vi "Enable All Disabled Programs.vi"(11 "EXID":u32=16773121 step=1 format="%.0x") -> ()   [LabVIEW 2010]
doc: "This VI Searches all device programs for programs that are defined AND disabled and re-enables them. This needs to be done to clear the device ActiveError byte."
uses:
  Drivers/Telemetry/Typedef Command List.ctl
panel:
  out "Affected Programs":string
  out "error out":errorcluster
  in  "error in (no error)":errorcluster
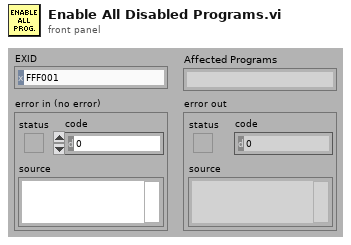
[diagram p1: front panel]
types:
  T1 = enum16{"Open Session", "Close Session", "Downlink Only", "Uplink Only", "Transceive (DN -> UP)"}
  T2 = typedef "Typedef Command List.ctl" = enum16{"Get xPG Status", "xPG Stimulation", "Select Program", "Increment Program Amplitude", "Decrement Program Amplitude", "Get PoP Constants", "Get PPC Constants", "Get Program Names", "Set Pulse Amplitude", "Increment Pulse Amplitude", "Decrement Pulse Amplitude", "Get Pulse Widths", "Set Pulse Widths", "Increment Pulse Width", "Decrement Pulse Width", "Get Program Frequency", "Set Program Frequency", "Increment Program Frequency", "Decrement Program Frequency", "Inject Event", "Charging Control", "Get xPG Identity", "Set xPG Identity", "Restore Program Defaults", "Get Program Definition", "Set Program Definition", "Get Program Constants", "Set Program Constants", "Get Configurable Device Parameters", "Set Configurable Device Parameters", "Get Pulse Constants", "Set Pulse Constants", "Get Lead Limits", "Set Lead Limits", "Get Channel Calibrations", "Set Channel Calibrations", "<reserved 2>", "<reserved 3>", "<reserved 4>", "<reserved 5>", "<reserved 6>", "<reserved 7>", "Get Stim Asic HV Calibrations", "Set Stim Asic HV Calibrations", "<reserved 8>", "<reserved 9>", "Get CP Data", "Set CP Data", "Clear Log", "Read Log", "Append Log", "Get Patient Program Runtime", "Set Patient Program Runtime", "Impedance Measurement", "Enter Storage Mode", "Echo Short", "Echo Long", "Get General Calibration", "Set General Calibration", "Get Trim List", "Set Trim List", "Get Counter", "Set Counter", "Get Test Stimulation", "Set Test Stimulation", "Get Titration Stimulation", "Set Titration Stimulation", "Get Ramp Time", "Set Ramp Time", "Get VBAT", "Set Software Description Block", "Get Software Description Block", "Write Memory", "Read Memory", "Reset xPG", "Erase Flash Block", "Write Vectors", "Read Vectors", "Diagnostic Data", "Set Background Impedance", "Get Background Impedence ", "Undefined"}
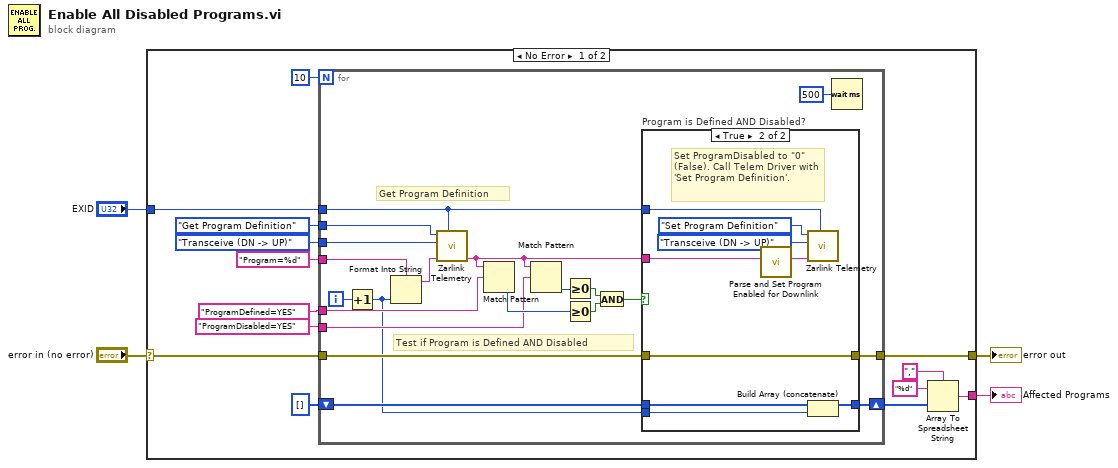
[diagram p0: block diagram]
diagram:
  n1 = case shown="No Error" "error in (no error)" {
    selector: "error in (no error)" -> [w13 w50]
    tunnel: [w12 w50] -> w3
    tunnel: [w6 _] -> w2
    tunnel: "EXID" -> [w5 _]
    frame No Error {
      n2 = for {
        N: 10 -> [_]
        tunnel: Typedef_Command_List."Get Program Definition" ("Command") -> [w38]
        tunnel: T1."Transceive (DN -> UP)" ("Function") -> [w37]
        tunnel: "Program=%d" -> [w35]
        tunnel: "ProgramDefined=YES" ("regular expression") -> [w33]
        tunnel: "ProgramDisabled=YES" ("regular expression") -> [w20]
        tunnel: w13 -> [w26]
        tunnel: [w25] -> w12
        shift-right: [w24] -> w9
        shift-left: i32[] [] -> [w23]
        tunnel: w5 -> [w21]
        i -> [w34]
        # "Test if Program is Defined AND Disabled"
        # "Get Program Definition"
        n3 = Increment(x=w34) -> (x+1=w19:i32)
        n4 = Format Into String(format string=w35, w19) -> (resulting string=w36:string)  [unwired: 2 in, 1 out]
        n5 = call "Zarlink Telemetry.vi"("EXID"=w21, "Parameters"=w36, "Function"=w37, "Command"=w38) -> ("Data"=w27:string)  [unwired: 2 in, 5 out]
        n6 = Match Pattern(string=w27, regular expression=w33) -> (offset past match=w32:i32)  [unwired: 1 in, 3 out]
        n7 = Match Pattern(string=w27, regular expression=w20) -> (offset past match=w31:i32)  [unwired: 1 in, 3 out]
        n8 = Greater Or Equal To 0?(x=w31) -> (x >= 0?=w29:bool)
        n9 = Greater Or Equal To 0?(x=w32) -> (x >= 0?=w30:bool)
        n10 = And(x=w29, y=w30) -> (x .and. y?=w28:bool)
        n11 = case "Program is Defined AND Disabled?" shown="True" w28 {
          tunnel: w27 -> [_ w43]
          tunnel: w26 -> [w40 w42]
          tunnel: [w40 w42] -> w25
          tunnel: w19 -> [_ w47]
          tunnel: [w39 w46] -> w24
          tunnel: w23 -> [w39 w45]
          tunnel: w21 -> [_ w44]
          frame False {
          }
          frame True {
            # "Set ProgramDisabled to \"0\" (False). Call Telem Driver with 'Set Program Definition'."
            n12 = call "Parse and Set Program Enabled for Downlink.vi"("Uplink String"=w43) -> ("Downlink String"=w41:string)  [unwired: 9 in]
            n13 = call "Zarlink Telemetry.vi"("EXID"=w44, "Parameters"=w41, "Function"=T1."Transceive (DN -> UP)", "Command"=Typedef_Command_List."Set Program Definition") -> ()  [unwired: 2 in, 6 out]
            n14 = Build Array (concatenate)(w45, w47) -> (w46:i32[])
          }
        }
        n15 = Wait (ms)(milliseconds to wait=u32 500) -> ()  [unwired: 1 out]
      }
      n16 = Array To Spreadsheet String(delimiter (Tab)=",", array=w9, 3:"%d") -> (spreadsheet string=w6:string)
    }
    frame Error {
    }
  }
  "error out" <- w3
  "Affected Programs" <- w2
